vi "Get MAC.vi"(8 "error in (no error)":errorcluster) -> (0 "error out":errorcluster, 2 "MAC addresses":string[][](array[string]), 3 "header":string[](array[string]))   [LabVIEW 2013]
panel:
  out "MAC addresses":i32(listbox)
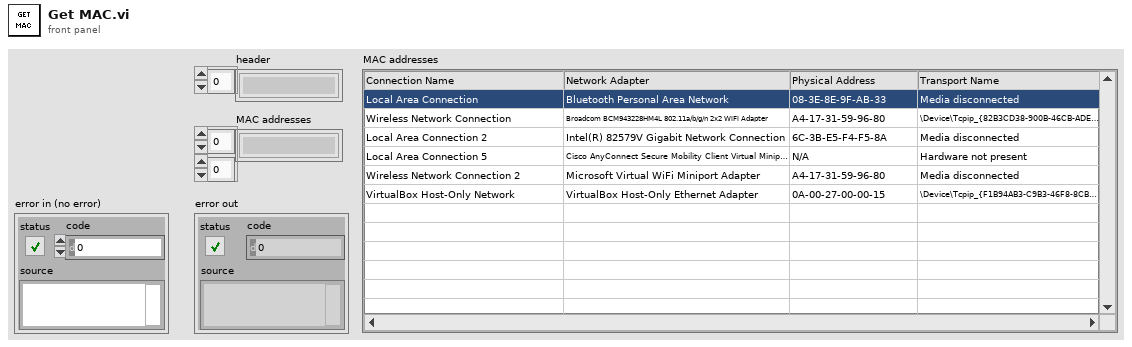
[diagram p1: front panel]
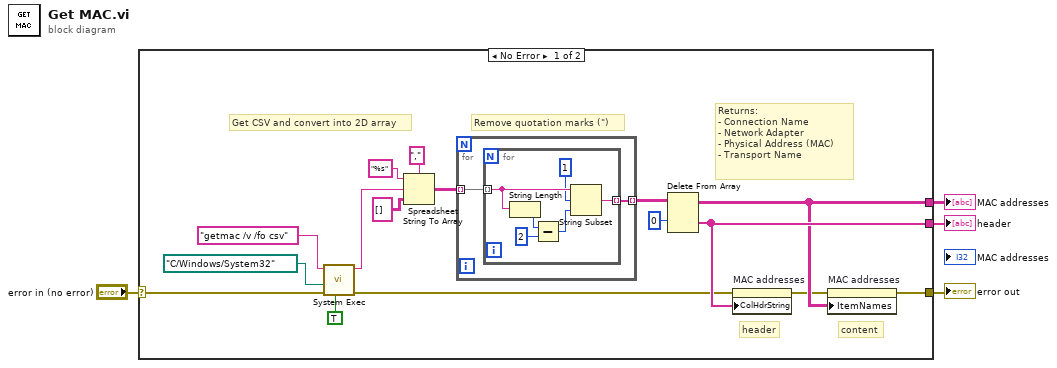
[diagram p0: block diagram]
diagram:
  n1 = case shown="No Error" "error in (no error)" {
    selector: "error in (no error)" -> [w8 w29]
    tunnel: [w12 _] -> w4
    tunnel: [w11 _] -> w3
    tunnel: [w5 w29] -> w2
    frame No Error {
      # "Get CSV and convert into 2D array"
      # "content"
      # "header"
      # "Remove quotation marks (\")"
      # "Returns:\n- Connection Name\n- Network Adapter\n- Physical Address (MAC)\n- Transport Name"
      n2 = call <vilib>:"System Exec.vi"("run minimized? (F)"=TRUE, "error in (no error)"=w8, "working directory"=path "C:/Windows/System32", "command line"="getmac /v /fo csv") -> ("error out"=w7:errorcluster, "standard output"=w14:string)  [unwired: 4 in, 2 out]
      n3 = Spreadsheet String To Array(delimiter (Tab)=",", format string="%s", spreadsheet string=w14, array type (2D Dbl)=string[][] []) -> (array=w10:string[][])
      n4 = for {
        tunnel: w10 -> [w22] mode=indexing
        tunnel: [w21] -> w9 mode=indexing
        n5 = for {
          tunnel: w22 -> [w28] mode=indexing
          tunnel: [w23] -> w21 mode=indexing
          n6 = String Length(string=w28) -> (length=w26:i32)
          n7 = Subtract(x=w26, y=2) -> (x-y=w27:i32)
          n8 = String Subset(string=w28, offset (0)=1, length (rest)=w27) -> (substring=w23:string)
        }
      }
      n9 = Delete From Array(array=w9, index (row)=0) -> (deleted portion=w12:string[], array with subset deleted=w11:string[][])  [unwired: 2 in]
      n10 = property on="MAC addresses" class="MCListbox (strict)"(error in=w7, "ColHdrString"=w12) -> (error out=w6:errorcluster)  [unwired: 1 in, 1 out]
      n11 = property on="MAC addresses" class="MCListbox (strict)"(error in=w6, "ItemNames"=w11) -> (error out=w5:errorcluster)  [unwired: 1 in, 1 out]
    }
    frame Error {
    }
  }
  "MAC addresses" <- w3
  "error out" <- w2
  "header" <- w4
